vi "SIM_Drive_Execute.vi"(5 "Initial Robot Position":T3 {"ROTATION"."SIN" format="%13.4f"; "ROTATION"."COS" format="%13.4f"; "ROTATION"."VALUE" format="%13.4f"; "TRANSLATION"."Y" format="%14.3f"; "TRANSLATION"."X" format="%14.3f"}, 6 "FPGA_Time_Seconds":dbl=-1.0, 7 "SwerveKinematics":T5 {"SavedModuleStates"."Angle"."SIN" format="%13.4f"; "SavedModuleStates"."Angle"."COS" format="%13.4f"; "SavedModuleStates"."Angle"."VALUE" format="%13.4f"; "PrevCoR"."Y" format="%14.3f"; "PrevCoR"."X" format="%14.3f"; "Modules"."Y" format="%14.3f"; "Modules"."X" format="%14.3f"}, 8 "in Module Positions":T1[](array[typedef]) {"Angle"."SIN" format="%13.4f"; "Angle"."COS" format="%13.4f"; "Angle"."VALUE" format="%13.4f"}, 9 "Battery Voltage":dbl, 10 "SpinMotorDmds":dbl[](array[numeric]), 11 "TravelMotorDmds":dbl[](array[numeric])) -> (0 "GyroStatus":T8, 1 "GyroValuesDeg":T9, 2 "out ModulePositions":T1[](array[typedef]) {"Angle"."SIN" format="%13.4f"; "Angle"."COS" format="%13.4f"; "Angle"."VALUE" format="%13.4f"}, 3 "ModuleStates":T7[](array[typedef]) {"Angle"."SIN" format="%13.4f"; "Angle"."COS" format="%13.4f"; "Angle"."VALUE" format="%13.4f"}, 4 "Motor Currents":dbl)   [LabVIEW 2023]
uses:
  <vilib>/Rock Robotics/WPI/ThirdParty/JAS_Junk/TrajLib/TypeDef/SWERVE_DRIVE_MODULE_STATE.ctl
  <vilib>/Rock Robotics/WPI/ThirdParty/JAS_Junk/TrajLib/TypeDef/ROTATION2D.ctl
  <vilib>/Rock Robotics/WPI/ThirdParty/JAS_Junk/TrajLib/TypeDef/SWERVE_DRIVE_MODULE_POSITION.ctl
  <vilib>/Rock Robotics/WPI/ThirdParty/ADI/ADIS16470/Typedef/ADIS16470 Data.ctl
  <vilib>/Rock Robotics/WPI/ThirdParty/ADI/ADIS16470/Typedef/ADIS16470 Status.ctl
  <vilib>/Rock Robotics/WPI/ThirdParty/JAS_Junk/TrajLib/TypeDef/SWERVE_DRIVE_KINEMATICS.ctl
  <vilib>/Analysis/Matrix/Datatypes/RealMatrix.ctl
  <vilib>/Rock Robotics/WPI/ThirdParty/JAS_Junk/TrajLib/TypeDef/TRANSLATION2D.ctl
  <vilib>/Rock Robotics/WPI/ThirdParty/JAS_Junk/TrajLib/TypeDef/POSE2D.ctl
  <vilib>/Rock Robotics/WPI/ThirdParty/JAS_Junk/TrajLib/VI/Util_GetTime_U32.vi
  <vilib>/Rock Robotics/WPI/ThirdParty/JAS_Junk/TrajLib/Conv_Radians_Deg.vi
  <vilib>/Rock Robotics/WPI/ThirdParty/JAS_Junk/TrajLib/VI/Util_GetTime_U64.vi
  SIM_Drive_Globals.vi
  <vilib>/Rock Robotics/WPI/ThirdParty/JAS_Junk/TrajLib/SwerveKinematics_ToChassisSpeedsX.vi
  <vilib>/Rock Robotics/WPI/ThirdParty/JAS_Junk/TrajLib/Trajectory_Library.lvlib
  <vilib>/Analysis/Matrix/NI_Matrix.lvlib
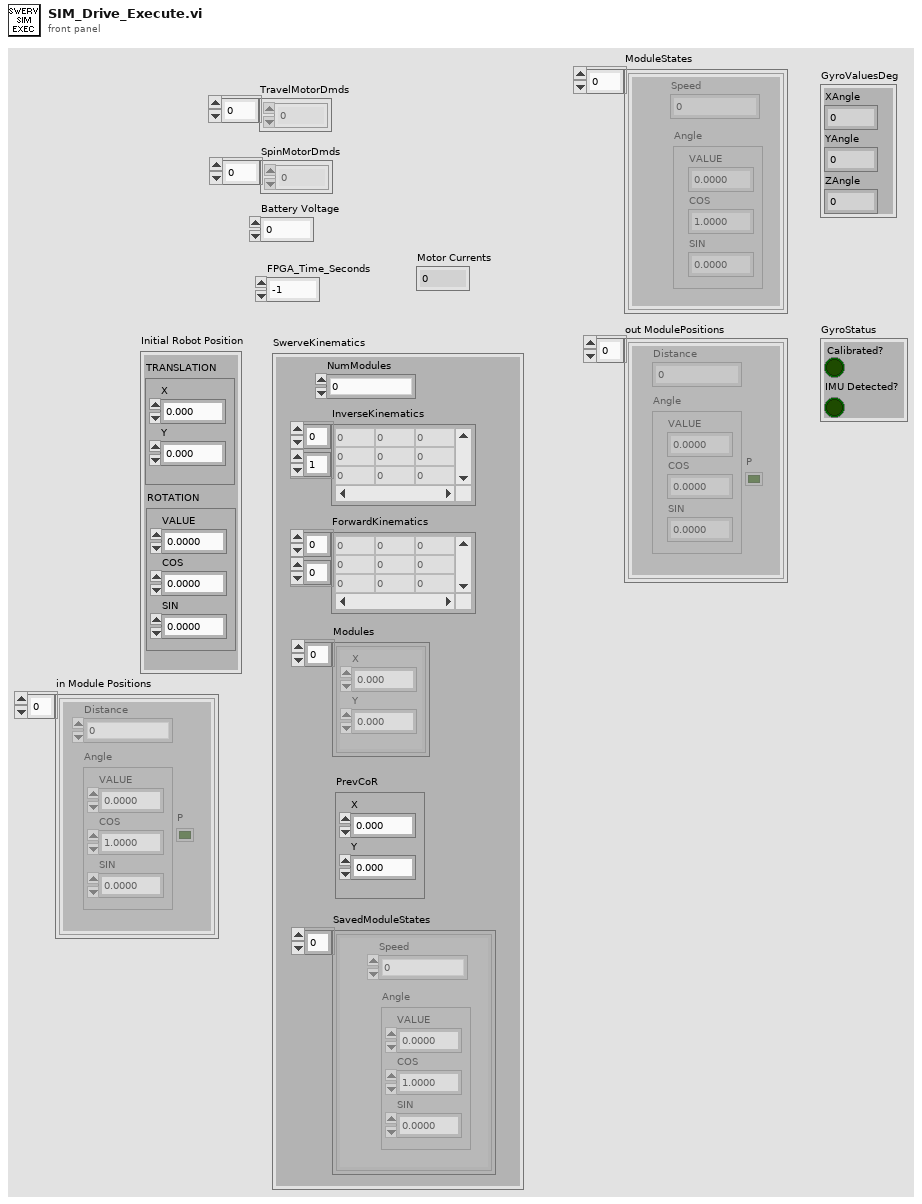
[diagram p1: front panel]
types:
  T1 = typedef "Trajectory_Library.lvlib/SWERVE_DRIVE_MODULE_POSITION.ctl" = cluster{"Distance":dbl, "Angle":T2, "P":bool}
  T2 = typedef "Trajectory_Library.lvlib/ROTATION2D.ctl" = cluster{"VALUE":dbl, "COS":dbl, "SIN":dbl}
  T3 = typedef "Trajectory_Library.lvlib/POSE2D.ctl" = cluster{"TRANSLATION":T4, "ROTATION":T2}
  T4 = typedef "Trajectory_Library.lvlib/TRANSLATION2D.ctl" = cluster{"X":dbl, "Y":dbl}
  T5 = typedef "Trajectory_Library.lvlib/SWERVE_DRIVE_KINEMATICS.ctl" = cluster{"NumModules":i32, "InverseKinematics":T6, "ForwardKinematics":T6, "Modules":T4[], "PrevCoR":T4, "SavedModuleStates":T7[]}
  T6 = typedef "NI_Matrix.lvlib/RealMatrix.ctl" = dbl[][]
  T7 = typedef "Trajectory_Library.lvlib/SWERVE_DRIVE_MODULE_STATE.ctl" = cluster{"Speed":dbl, "Angle":T2}
  T8 = typedef "ADIS16470 Status.ctl" = cluster{"Calibrated?":bool, "IMU Detected?":bool}
  T9 = typedef "ADIS16470 Data.ctl" = cluster{"XAngle":dbl, "YAngle":dbl, "ZAngle":dbl}
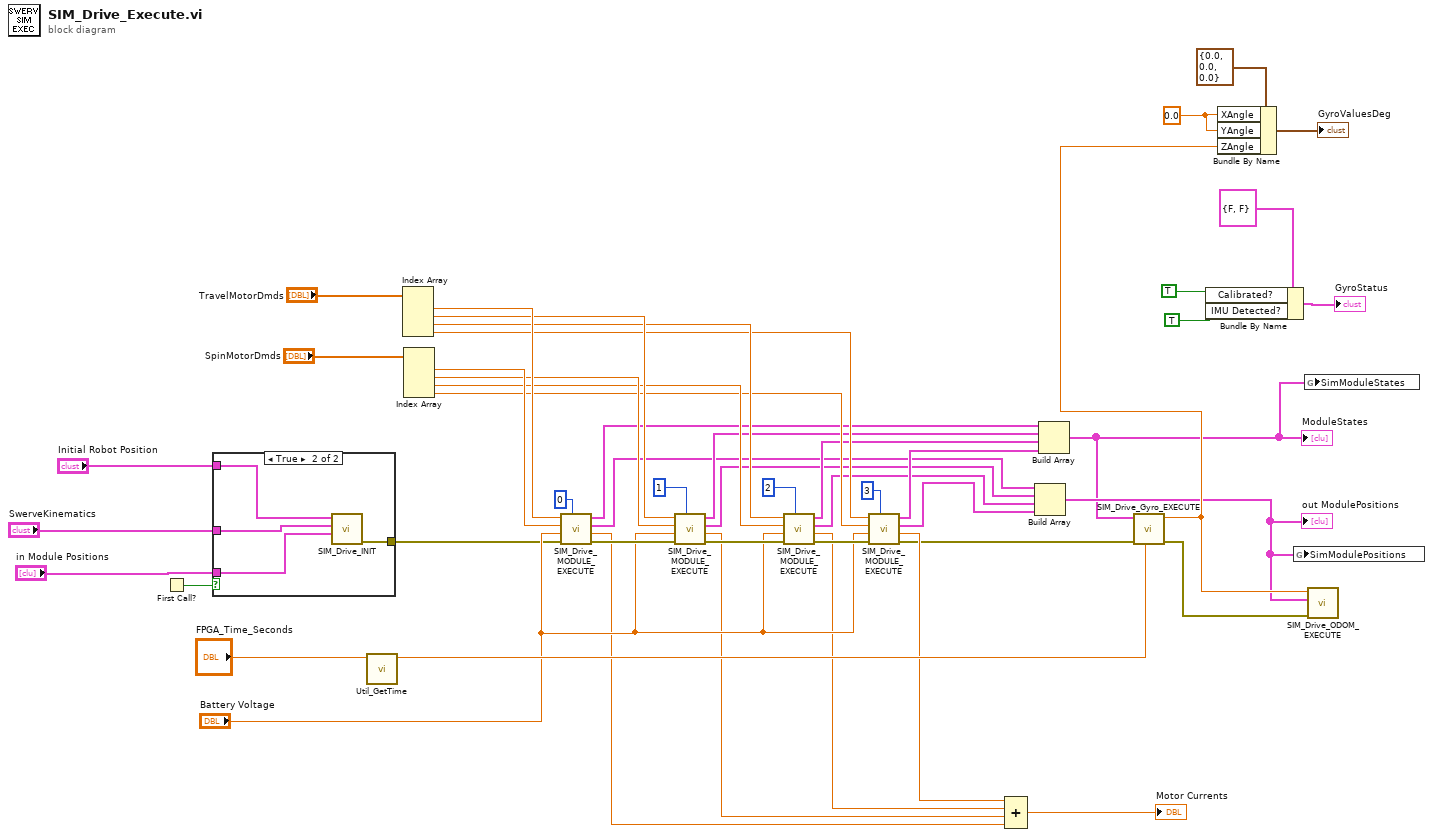
[diagram p0: block diagram]
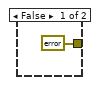
[diagram p2: hidden frame]
diagram:
  w22 = 0.0 ("YAngle")
  n1 = First Call?() -> (First Call?: T/F=w35:bool)
  n2 = case shown="True" w35 {
    tunnel: [errorcluster {"status"=FALSE, "code"=0, "source"=""} ("error out") w55] -> w2
    tunnel: "Initial Robot Position" -> [_ w54]
    tunnel: "SwerveKinematics" -> [_ w53]
    tunnel: "in Module Positions" -> [_ w52]
    frame False {
    }
    frame True {
      n3 = call "SIM_Drive_INIT.vi"("Module Positions"=w52, "Simulation_Kinematics"=w53, "Initial Robot Position"=w54) -> ("error out"=w55:errorcluster)  [unwired: 8 in]
    }
  }
  n4 = call <vilib>:"Util_GetTime.vi"("Pass_Through_Time"="FPGA_Time_Seconds") -> ("FPGA_Time_Seconds"=w42:dbl)  [unwired: 8 in, 2 out]
  n5 = Index Array(array="TravelMotorDmds") -> (element #1=w32:dbl, element #2=w30:dbl, element #3=w28:dbl, element #4=w26:dbl)  [unwired: 4 in]
  n6 = Index Array(array="SpinMotorDmds") -> (element #1=w31:dbl, element #2=w29:dbl, element #3=w27:dbl, element #4=w25:dbl)  [unwired: 4 in]
  n7 = call "SIM_Drive_MODULE_EXECUTE.vi"("Module Index"=0, "error in (no error)"=w2, "Battery Voltage"="Battery Voltage", "SpinMotorDmd"=w31, "TravelMotorDmd"=w32) -> ("error out"=w49:errorcluster, "Abs Current"=w37:dbl, "ModulePosition"=w13:T1, "ModuleState"=w17:T7)  [unwired: 3 in]
  n8 = call "SIM_Drive_MODULE_EXECUTE.vi"("Module Index"=1, "error in (no error)"=w49, "Battery Voltage"="Battery Voltage", "SpinMotorDmd"=w29, "TravelMotorDmd"=w30) -> ("error out"=w48:errorcluster, "Abs Current"=w38:dbl, "ModulePosition"=w12:T1, "ModuleState"=w16:T7)  [unwired: 3 in]
  n9 = call "SIM_Drive_MODULE_EXECUTE.vi"("Module Index"=2, "error in (no error)"=w48, "Battery Voltage"="Battery Voltage", "SpinMotorDmd"=w27, "TravelMotorDmd"=w28) -> ("error out"=w47:errorcluster, "Abs Current"=w39:dbl, "ModulePosition"=w11:T1, "ModuleState"=w15:T7)  [unwired: 3 in]
  n10 = call "SIM_Drive_MODULE_EXECUTE.vi"("Module Index"=3, "error in (no error)"=w47, "Battery Voltage"="Battery Voltage", "SpinMotorDmd"=w25, "TravelMotorDmd"=w26) -> ("error out"=w4:errorcluster, "Abs Current"=w40:dbl, "ModulePosition"=w10:T1, "ModuleState"=w14:T7)  [unwired: 3 in]
  n11 = Compound Arithmetic op=ADD(w40, w39, w38, w37) -> (→"Motor Currents":dbl)
  n12 = Build Array(w13, w12, w11, w10) -> (w8:T1[])
  "out ModulePositions" <- w8
  n13 = Build Array(w17, w16, w15, w14) -> (w1:T7[])
  "ModuleStates" <- w1
  n14 = call "SIM_Drive_Gyro_EXECUTE.vi"("FPGA_Time_Seconds"=w42, "error in (no error)"=w4, "ModuleStates"=w1) -> ("error out"=w3:errorcluster, "GyroYawDegrees"=w9:dbl)  [unwired: 7 in]
  n15 = Bundle By Name(cluster=T8 {"Calibrated?"=FALSE, "IMU Detected?"=FALSE} ("GyroStatus"), "Calibrated?"=TRUE ("IMU Detected?"), "IMU Detected?"=TRUE) -> (→"GyroStatus":T8)
  n16 = Bundle By Name(cluster=T9 {"XAngle"=0.0, "YAngle"=0.0, "ZAngle"=0.0} ("GyroValuesDeg"), "XAngle"=w22, "YAngle"=w22, "ZAngle"=w9) -> (→"GyroValuesDeg":T9)
  n17 = global write "SIM_Drive_Globals.vi" "SimModulePositions"(w8) -> ()
  n18 = global write "SIM_Drive_Globals.vi" "SimModuleStates"(w1) -> ()
  n19 = call "SIM_Drive_ODOM_EXECUTE.vi"("error in (no error)"=w3, "module Positions"=w8, "GyroAngleDeg"=w9) -> ()  [unwired: 8 in, 1 out]
